vi "SeqLoop.vi"(6 "SEQ STEP Display":refnum<notifier>, 8 "error in (no error)":errorcluster, 9 "SEQ":refnum<queue>, 10 "CORE":refnum<queue>, 11 "WINFAS 2 Data Queue":T1) -> (0 "error out":errorcluster)   [LabVIEW 2014, in "SeqLoop.lvlib"]
uses:
  SeqLoop.lvlib
  APIs/Message Queue/Message Cluster.ctl
  APIs/Data Queue/All Data Queues Cluster.ctl
  APIs/Data Queue/Acquisition Data 1 Sample Cluster.ctl
  APIs/Data Queue/Control Data Cluster.ctl
  APIs/Data Queue/Async Acquisition Data Cluster.ctl
  TypeDefs/STEP Display.ctl
  Mimico Display/TypeDefs/Mimic Data.ctl
  Mimico Display/TypeDefs/BG Image.ctl
  Mimico Display/TypeDefs/mObject.ctl
  TypeDefs/Program.ctl
  TypeDefs/Sequence.ctl
  TypeDefs/STEP.ctl
  TypeDefs/LogicParsedExpression.ctl
  TypeDefs/HW InOut MAP.ctl
  TypeDefs/HW Variables State.ctl
  TypeDefs/STEP State.ctl
  APIs/Message Queue/Enqueue Message (Single).vi
  SEQ Monitoring Global Variables.vi
  APIs/Message Queue/WINFAS 2 Message Queue.lvlib
  Mimico Display/Mimico Display.lvlib
  APIs/Data Queue/WINFAS 2 Data Queue.lvlib
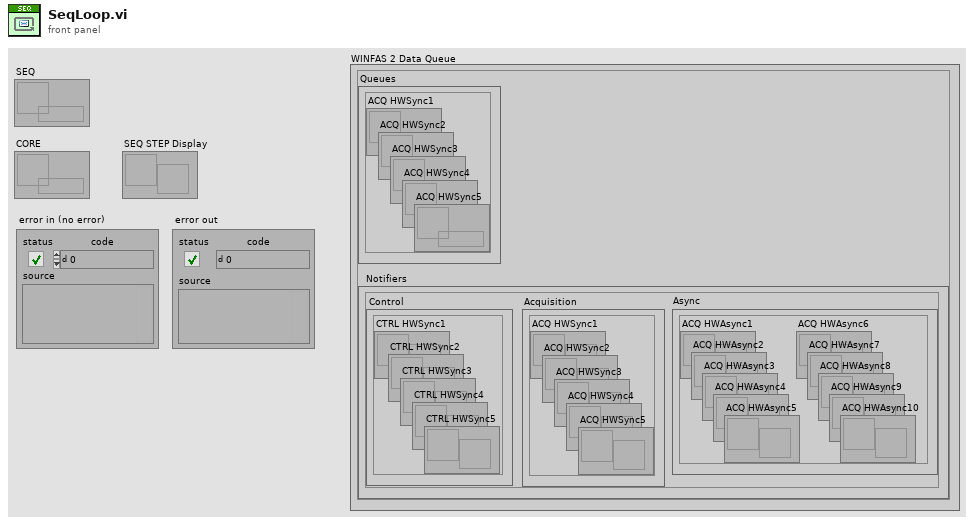
[diagram p1: front panel]
types:
  T1 = typedef "WINFAS 2 Data Queue.lvlib/All Data Queues Cluster.ctl" = cluster{"Queues":cluster{"ACQ HWSync1":refnum<queue>, "ACQ HWSync2":refnum<queue>, "ACQ HWSync3":refnum<queue>, "ACQ HWSync4":refnum<queue>, "ACQ HWSync5":refnum<queue>}, "Notifiers":cluster{"Control":cluster{"CTRL HWSync1":refnum<notifier>, "CTRL HWSync2":refnum<notifier>, "CTRL HWSync3":refnum<notifier>, "CTRL HWSync4":refnum<notifier>, "CTRL HWSync5":refnum<notifier>}, "Acquisition":cluster{"ACQ HWSync1":refnum<notifier>, "ACQ HWSync2":refnum<notifier>, "ACQ HWSync3":refnum<notifier>, "ACQ HWSync4":refnum<notifier>, "ACQ HWSync5":refnum<notifier>}, "Async":cluster{"ACQ HWAsync1":refnum<notifier>, "ACQ HWAsync2":refnum<notifier>, "ACQ HWAsync3":refnum<notifier>, "ACQ HWAsync4":refnum<notifier>, "ACQ HWAsync5":refnum<notifier>, "ACQ HWAsync6":refnum<notifier>, "ACQ HWAsync7":refnum<notifier>, "ACQ HWAsync8":refnum<notifier>, "ACQ HWAsync9":refnum<notifier>, "ACQ HWAsync10":refnum<notifier>}}}
  T2 = typedef "SeqLoop.lvlib/Sequence.ctl" = cluster{"STEPs":T3[], "Main Error&Alarm":cluster{"Main Error":T4, "Main Alarm 1":T4, "Main Alarm 2":T4, "Main Alarm 3":T4, "Main Alarm 4":T4}}
  T3 = typedef "SeqLoop.lvlib/STEP.ctl" = cluster{"STEP N°":u32, "STEP Switch":cluster{"jump?":bool, "Initial STEP":u32, "Number of STEPs":u32, "Repetitions":u32, "Reset?":bool}, "Outputs":i32[], "STEP Check":cluster{"Advance":T4, "Error ":T4, "Alarm 1":T4, "Alarm 2":T4, "Alarm 3":T4, "Alarm 4":T4}, "Display":cluster{"Mssg Op":string, "Mimic Data":T5}}
  T4 = typedef "SeqLoop.lvlib/LogicParsedExpression.ctl" = cluster{"RPN ":string[], "Variables":string[], "Ctes":string[], "Formula":string, "Message":string}
  T5 = typedef "SeqLoop.lvlib/Mimico Display.lvlib/Mimic Data.ctl" = cluster{"BG Image":T6, "Mimic mObjects":T7[]}
  T6 = typedef "SeqLoop.lvlib/Mimico Display.lvlib/BG Image.ctl" = cluster{"Path":path, "point":cluster{"x":i16, "y":i16}}
  T7 = typedef "SeqLoop.lvlib/Mimico Display.lvlib/mObject.ctl" = cluster{"point":cluster{"x":i16, "y":i16}, "Precision (Digits)":i32, "Visible?":bool, "Ref":string, "Comment":string}
  T8 = typedef "SeqLoop.lvlib/STEP State.ctl" = enum16{"Stopped", "First Call", "Idle...", "Advance OK", "Alarm", "Output Security", "Error"}
  T9 = typedef "SeqLoop.lvlib/HW Variables State.ctl" = cluster{"I":bool[], "P":bool[], "N":bool[], "T":bool[], "X":bool[], "Timer":u32[], "Wait":u32, "Wait?":bool, "Jump":cluster{"Jumping?":bool, "Previous STEP to Jump":u32, "Initial Jump STEP":u32, "STEP Count":u32, "Loop Count":u32, "Number of STEPs":u32, "Repetitions":u32}, "Reset?":bool}
  T10 = typedef "SeqLoop.lvlib/HW InOut MAP.ctl" = cluster{"Inputs":cluster{"Entrada":i32, "Descripción":string, "Habilitada?":bool}[][], "Outputs":cluster{"Salida":i32, "Descripción":string, "Habilitada?":bool, "Formula":string, "Tipo de Salida":string}[][]}
  T11 = typedef "SeqLoop.lvlib/Program.ctl" = cluster{"Prog. Data":cluster{"Operación":i32, "Pieza":i32, "Descripción":string, "Nombre Programa":string, "Autor":string, "Diseño":string, "Total Meds.:":i32, "Total Meds. Aux.:":i32}, "All Sequences":cluster{"Measurement":T2, "AutoZero":T2}}
  T12 = cluster{"CTRL HWSync1":refnum<notifier>, "CTRL HWSync2":refnum<notifier>, "CTRL HWSync3":refnum<notifier>, "CTRL HWSync4":refnum<notifier>, "CTRL HWSync5":refnum<notifier>}
  T13 = cluster{"File Direction":path, "Progs Data":variant}
  T14 = typedef "SeqLoop.lvlib/HW CTRL Data.ctl" = cluster{"Inputs":bool[], "Encoder 1":sgl, "Encoder 2":sgl, "Encoder 3":sgl, "Encoder 4":sgl, "Encoder 5":sgl}
  T15 = cluster{"Alarm 1":bool, "Alarm 2":bool, "Alarm 3":bool, "Alarm 4":bool, "Main Err&Alarm?":bool}
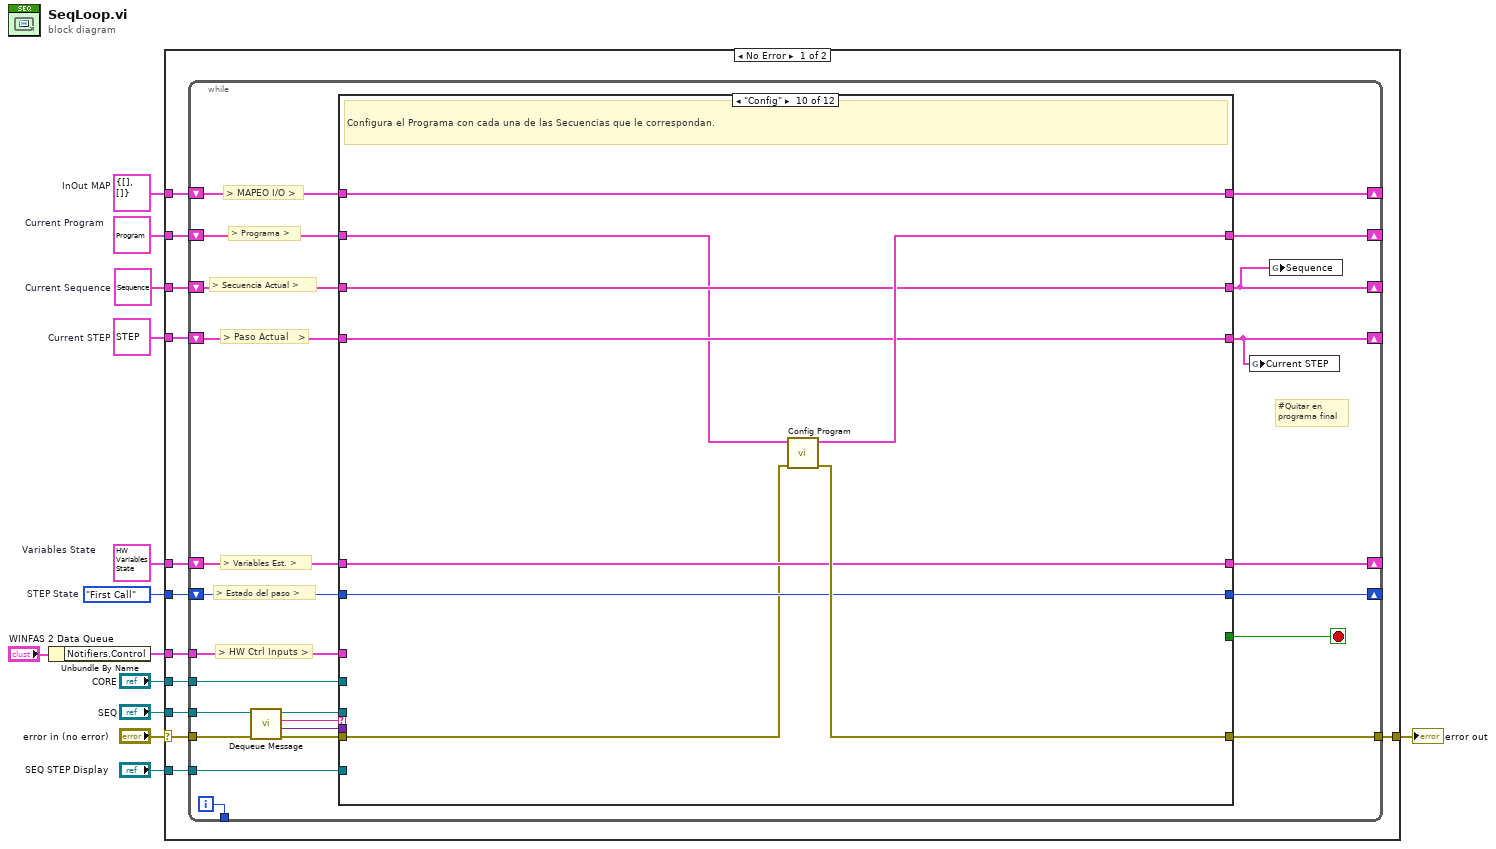
[diagram p0: block diagram]
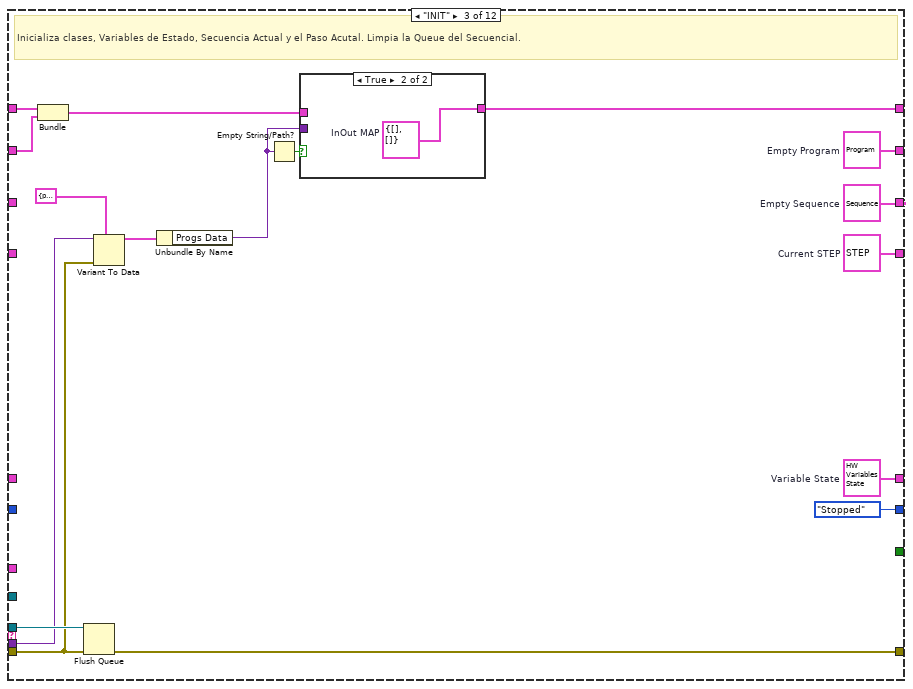
[diagram p4: hidden frame]
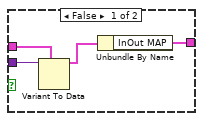
[diagram p5: hidden frame]
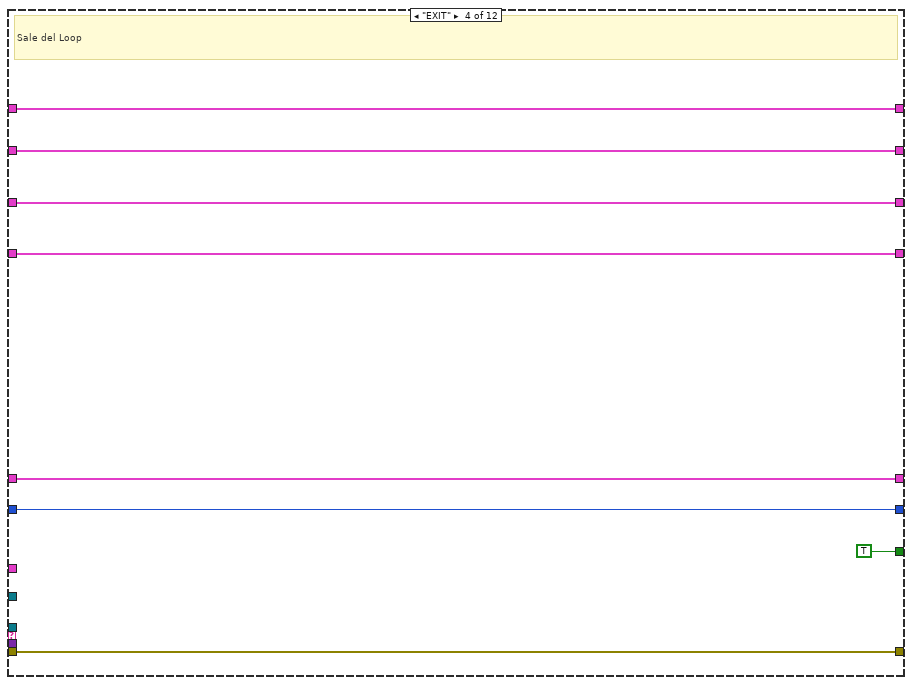
[diagram p6: hidden frame]
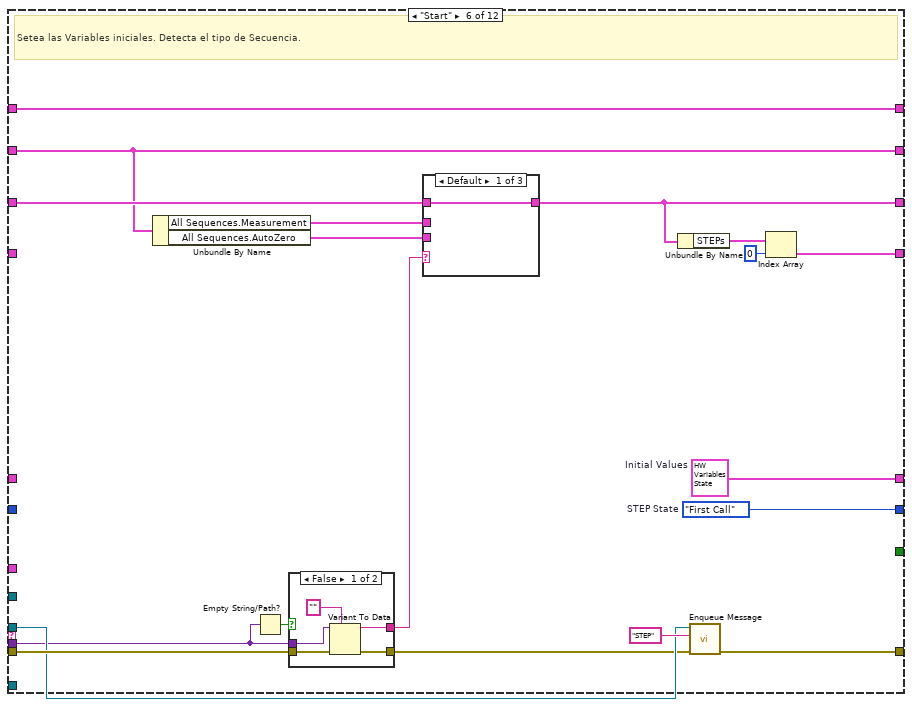
[diagram p8: hidden frame]
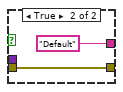
[diagram p9: hidden frame]
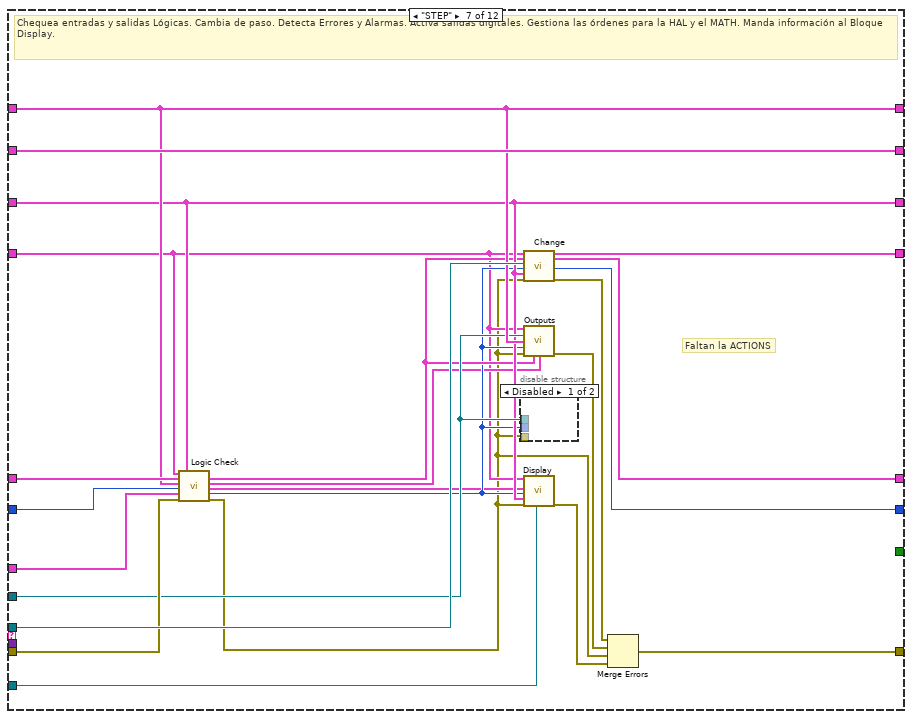
[diagram p12: hidden frame]
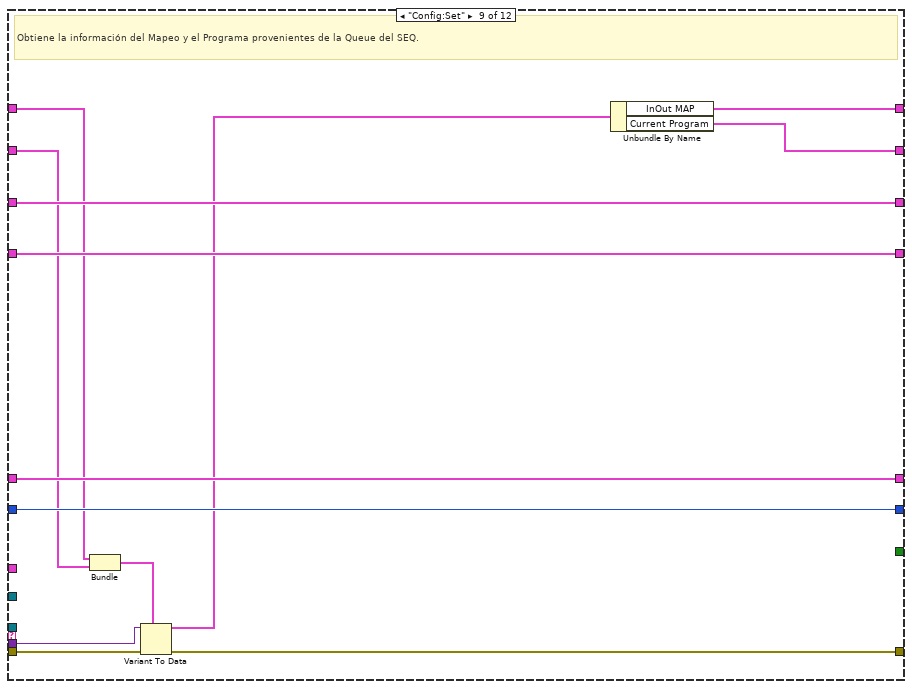
[diagram p15: hidden frame]
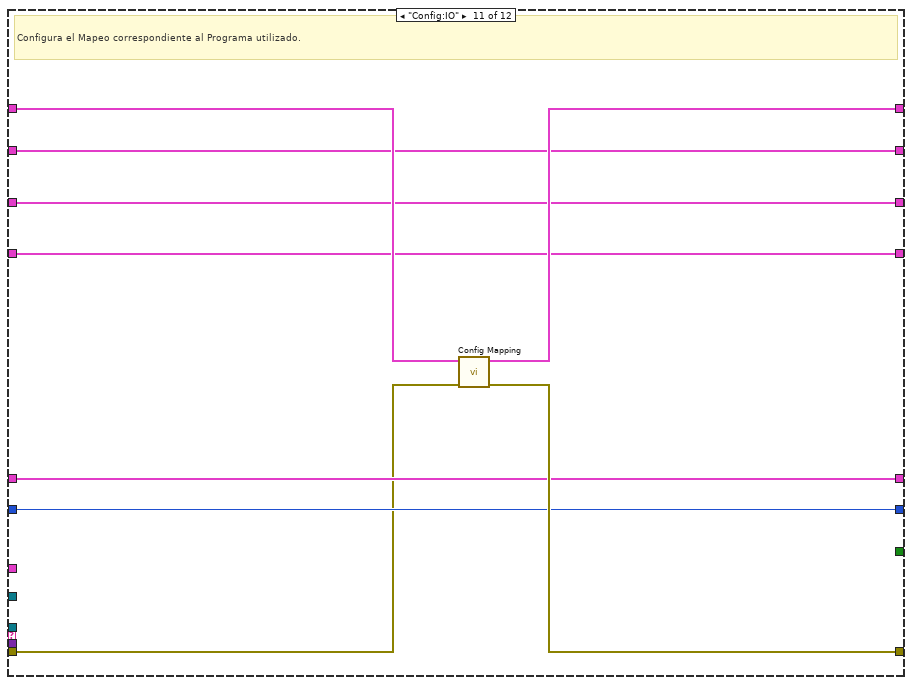
[diagram p16: hidden frame]
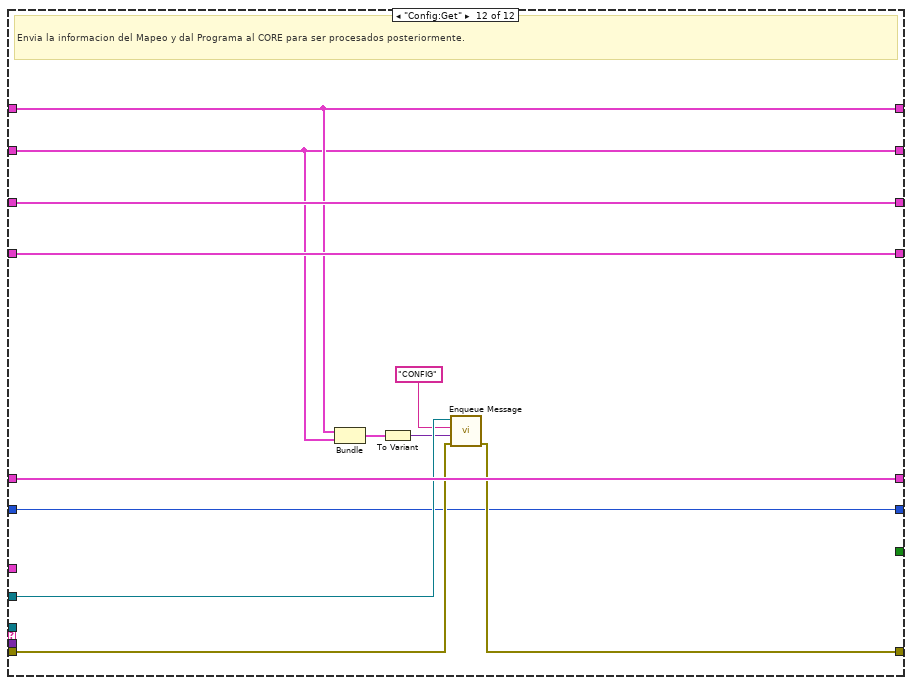
[diagram p17: hidden frame]
diagram:
  w2 = T2 {"STEPs"=[], "Main Error&Alarm"={"Main Error"={"RPN "=[], "Variables"=[], "Ctes"=[], "Formula"="", "Message"=""}, "Main Alarm 1"={"RPN "=[], "Variables"=[], "Ctes"=[], "Formula"="", "Message"=""}, "Main Alarm 2"={"RPN "=[], "Variables"=[], "Ctes"=[], "Formula"="", "Message"=""}, "Main Alarm 3"={"RPN "=[], "Variables"=[], "Ctes"=[], "Formula"="", "Message"=""}, "Main Alarm 4"={"RPN "=[], "Variables"=[], "Ctes"=[], "Formula"="", "Message"=""}}}  # Current Sequence
  w1 = T3 {"STEP N°"=0, "STEP Switch"={"jump?"=FALSE, "Initial STEP"=0, "Number of STEPs"=0, "Repetitions"=0, "Reset?"=FALSE}, "Outputs"=[], "STEP Check"={"Advance"={"RPN "=[], "Variables"=[], "Ctes"=[], "Formula"="", "Message"=""}, "Error "={"RPN "=[], "Variables"=[], "Ctes"=[], "Formula"="", "Message"=""}, "Alarm 1"={"RPN "=[], "Variables"=[], "Ctes"=[], "Formula"="", "Message"=""}, "Alarm 2"={"RPN "=[], "Variables"=[], "Ctes"=[], "Formula"="", "Message"=""}, "Alarm 3"={"RPN "=[], "Variables"=[], "Ctes"=[], "Formula"="", "Message"=""}, "Alarm 4"={"RPN "=[], "Variables"=[], "Ctes"=[], "Formula"="", "Message"=""}}, "Display"={"Mssg Op"="", "Mimic Data"={"BG Image"={"Path"=path "", "point"={"x"=0, "y"=0}}, "Mimic mObjects"=[]}}}  # Current STEP
  w6 = STEP_State."First Call"  # STEP State
  w7 = T9 {"I"=[], "P"=[], "N"=[], "T"=[], "X"=[], "Timer"=[], "Wait"=0, "Wait?"=FALSE, "Jump"={"Jumping?"=FALSE, "Previous STEP to Jump"=0, "Initial Jump STEP"=0, "STEP Count"=0, "Loop Count"=0, "Number of STEPs"=0, "Repetitions"=0}, "Reset?"=FALSE}  # Variables State
  w9 = T10 {"Inputs"=[], "Outputs"=[]}  # InOut MAP
  w8 = T11 {"Prog. Data"={"Operación"=0, "Pieza"=0, "Descripción"="", "Nombre Programa"="", "Autor"="", "Diseño"="", "Total Meds.:"=0, "Total Meds. Aux.:"=0}, "All Sequences"={"Measurement"={"STEPs"=[], "Main Error&Alarm"={"Main Error"={"RPN "=[], "Variables"=[], "Ctes"=[], "Formula"="", "Message"=""}, "Main Alarm 1"={"RPN "=[], "Variables"=[], "Ctes"=[], "Formula"="", "Message"=""}, "Main Alarm 2"={"RPN "=[], "Variables"=[], "Ctes"=[], "Formula"="", "Message"=""}, "Main Alarm 3"={"RPN "=[], "Variables"=[], "Ctes"=[], "Formula"="", "Message"=""}, "Main Alarm 4"={"RPN "=[], "Variables"=[], "Ctes"=[], "Formula"="", "Message"=""}}}, "AutoZero"={"STEPs"=[], "Main Error&Alarm"={"Main Error"={"RPN "=[], "Variables"=[], "Ctes"=[], "Formula"="", "Message"=""}, "Main Alarm 1"={"RPN "=[], "Variables"=[], "Ctes"=[], "Formula"="", "Message"=""}, "Main Alarm 2"={"RPN "=[], "Variables"=[], "Ctes"=[], "Formula"="", "Message"=""}, "Main Alarm 3"={"RPN "=[], "Variables"=[], "Ctes"=[], "Formula"="", "Message"=""}, "Main Alarm 4"={"RPN "=[], "Variables"=[], "Ctes"=[], "Formula"="", "Message"=""}}}}}  # Current Program
  n1 = Unbundle By Name("WINFAS 2 Data Queue") -> ("Notifiers.Control"=w4:T12)
  n2 = case shown="No Error" "error in (no error)" {
    selector: "error in (no error)" -> [w25 w203]
    tunnel: [w18 w203] -> w12
    tunnel: "CORE" -> [w24 _]
    tunnel: "SEQ" -> [w23 _]
    tunnel: w9 -> [w22 _]
    tunnel: w8 -> [w21 _]
    tunnel: w2 -> [w17 _]
    tunnel: w7 -> [w20 _]
    tunnel: "SEQ STEP Display" -> [w19 _]
    tunnel: w6 -> [w16 _]
    tunnel: w4 -> [w15 _]
    tunnel: w1 -> [w14 _]
    frame No Error {
      n3 = while {
        tunnel: w25 -> [w45]
        tunnel: [w33] -> w18
        tunnel: w23 -> [w46]
        shift-right: [w47] -> _
        shift-left: w20 -> [w48]
        shift-right: [w40] -> _
        shift-left: w22 -> [w41]
        shift-right: [w38] -> _
        shift-left: w21 -> [w39]
        tunnel: w24 -> [w37]
        tunnel: w19 -> [w36]
        shift-right: [w28] -> _
        shift-left: w17 -> [w34]
        tunnel: w15 -> [w35]
        shift-right: [w26] -> _
        shift-left: w14 -> [w30]
        shift-right: [w29] -> _
        shift-left: w16 -> [w31]
        tunnel: [w27] -> _
        i -> [w27]
        stop <- w49 stop-if-true
        # "#Quitar en\nprograma final"
        # "> HW Ctrl Inputs >"
        # "> Variables Est. >"
        # "> Estado del paso >"
        # "> Paso Actual   >"
        # "> Secuencia Actual >"
        # "> Programa >"
        # "> MAPEO I/O >"
        n4 = call "Dequeue Message.vi"("error in (no error)"=w45, "Message Queue"=w46) -> ("error out"=w44:errorcluster, "Message Data"=w42:variant, "Message"=w43:string, "dup Message Queue"=w32:refnum<queue>)  [unwired: 6 in]
        n5 = case shown="\"Config\"" w43 {
          tunnel: [w55 w59 w78 w91 w100 w111 w147 w158 w161 w181 w190 w199] -> w33
          tunnel: w44 -> [w55 w59 w76 w91 w100 w117 w142 w158 w171 w174 w182 w200]
          tunnel: w42 -> [_ _ w75 _ _ w102 _ _ w170 _ _ _]
          tunnel: [_ _ _ TRUE _ _ _ _ _ _ _ _] -> w49
          tunnel: w48 -> [w56 w63 _ w92 w99 _ w145 w159 w172 w180 w189 w202]
          tunnel: [w56 w63 w79 w92 w99 w109 w137 w159 w172 w180 w189 w202] -> w47
          tunnel: w41 -> [w52 w61 w72 w88 w97 w115 w141 w155 w164 w179 w188 w193]
          tunnel: [w52 w61 w70 w88 w97 w115 w141 w155 w167 w179 w187 w193] -> w40
          tunnel: w39 -> [w54 w62 w71 w90 w98 w112 w150 w157 w163 w173 w186 w192]
          tunnel: [w54 w62 w65 w90 w98 w112 w150 w157 w168 w178 w186 w192] -> w38
          tunnel: w37 -> [_ _ _ _ _ _ w140 _ _ _ _ w201]
          tunnel: w36 -> [_ _ _ _ _ _ w144 _ _ _ _ _]
          tunnel: [w53 w60 w64 w89 w96 w105 w136 w156 w169 w177 w185 w197] -> w28
          tunnel: w34 -> [w53 w60 _ w89 w96 w113 w136 w156 w169 w177 w185 w197]
          tunnel: w35 -> [_ _ _ _ _ _ w146 _ _ _ _ _]
          tunnel: w32 -> [_ _ w80 _ _ w114 w148 _ _ _ _ _]
          tunnel: w31 -> [w50 w57 _ w86 w94 _ w143 w153 w165 w175 w183 w195]
          tunnel: [w51 w58 w67 w87 w95 w103 w151 w154 w166 w176 w184 w196] -> w26
          tunnel: w30 -> [w51 w58 _ w87 w95 _ w131 w154 w166 w176 w184 w196]
          tunnel: [w50 w57 STEP_State."Stopped" ("STEP State") w86 w94 w107 w149 w153 w165 w175 w183 w195] -> w29
          frame "----LOOP----" {
            # "Bloque que adminte futuras configuraciones al inicio."
          }
          frame Default {
          }
          frame "INIT" {
            w64 = T2 {"STEPs"=[], "Main Error&Alarm"={"Main Error"={"RPN "=[], "Variables"=[], "Ctes"=[], "Formula"="", "Message"=""}, "Main Alarm 1"={"RPN "=[], "Variables"=[], "Ctes"=[], "Formula"="", "Message"=""}, "Main Alarm 2"={"RPN "=[], "Variables"=[], "Ctes"=[], "Formula"="", "Message"=""}, "Main Alarm 3"={"RPN "=[], "Variables"=[], "Ctes"=[], "Formula"="", "Message"=""}, "Main Alarm 4"={"RPN "=[], "Variables"=[], "Ctes"=[], "Formula"="", "Message"=""}}}  # Empty Sequence
            w67 = T3 {"STEP N°"=0, "STEP Switch"={"jump?"=FALSE, "Initial STEP"=0, "Number of STEPs"=0, "Repetitions"=0, "Reset?"=FALSE}, "Outputs"=[], "STEP Check"={"Advance"={"RPN "=[], "Variables"=[], "Ctes"=[], "Formula"="", "Message"=""}, "Error "={"RPN "=[], "Variables"=[], "Ctes"=[], "Formula"="", "Message"=""}, "Alarm 1"={"RPN "=[], "Variables"=[], "Ctes"=[], "Formula"="", "Message"=""}, "Alarm 2"={"RPN "=[], "Variables"=[], "Ctes"=[], "Formula"="", "Message"=""}, "Alarm 3"={"RPN "=[], "Variables"=[], "Ctes"=[], "Formula"="", "Message"=""}, "Alarm 4"={"RPN "=[], "Variables"=[], "Ctes"=[], "Formula"="", "Message"=""}}, "Display"={"Mssg Op"="", "Mimic Data"={"BG Image"={"Path"=path "", "point"={"x"=0, "y"=0}}, "Mimic mObjects"=[]}}}  # Current STEP
            w65 = T11 {"Prog. Data"={"Operación"=0, "Pieza"=0, "Descripción"="", "Nombre Programa"="", "Autor"="", "Diseño"="", "Total Meds.:"=0, "Total Meds. Aux.:"=0}, "All Sequences"={"Measurement"={"STEPs"=[], "Main Error&Alarm"={"Main Error"={"RPN "=[], "Variables"=[], "Ctes"=[], "Formula"="", "Message"=""}, "Main Alarm 1"={"RPN "=[], "Variables"=[], "Ctes"=[], "Formula"="", "Message"=""}, "Main Alarm 2"={"RPN "=[], "Variables"=[], "Ctes"=[], "Formula"="", "Message"=""}, "Main Alarm 3"={"RPN "=[], "Variables"=[], "Ctes"=[], "Formula"="", "Message"=""}, "Main Alarm 4"={"RPN "=[], "Variables"=[], "Ctes"=[], "Formula"="", "Message"=""}}}, "AutoZero"={"STEPs"=[], "Main Error&Alarm"={"Main Error"={"RPN "=[], "Variables"=[], "Ctes"=[], "Formula"="", "Message"=""}, "Main Alarm 1"={"RPN "=[], "Variables"=[], "Ctes"=[], "Formula"="", "Message"=""}, "Main Alarm 2"={"RPN "=[], "Variables"=[], "Ctes"=[], "Formula"="", "Message"=""}, "Main Alarm 3"={"RPN "=[], "Variables"=[], "Ctes"=[], "Formula"="", "Message"=""}, "Main Alarm 4"={"RPN "=[], "Variables"=[], "Ctes"=[], "Formula"="", "Message"=""}}}}}  # Empty Program
            w79 = T9 {"I"=[], "P"=[], "N"=[], "T"=[], "X"=[], "Timer"=[], "Wait"=0, "Wait?"=FALSE, "Jump"={"Jumping?"=FALSE, "Previous STEP to Jump"=0, "Initial Jump STEP"=0, "STEP Count"=0, "Loop Count"=0, "Number of STEPs"=0, "Repetitions"=0}, "Reset?"=FALSE}  # Variable State
            # "Inicializa clases, Variables de Estado, Secuencia Actual y el Paso Acutal. Limpia la Queue del Secuencial."
            n6 = Bundle("InOut MAP"=w72, "Current Program"=w71) -> (w73:cluster{"InOut MAP":T10, "Current Program":T11})  [unwired: 1 in]
            n7 = Flush Queue(queue=w80, error in (no error)=w76) -> (error out=w78:errorcluster)  [unwired: 2 out]
            n8 = Variant To Data(error in=w76, type=T13 {"File Direction"=path "", "Progs Data"=variant} ("element"), Variant=w75) -> (data=w74:T13)  [unwired: 1 out]
            n9 = Unbundle By Name(w74) -> ("Progs Data"=w69:variant)
            n10 = Empty String/Path?(string/path=w69) -> (empty?=w68:bool)
            n11 = case shown="True" w68 {
              tunnel: w73 -> [w84 _]
              tunnel: [w82 w85] -> w70
              tunnel: w69 -> [w81 _]
              frame False {
                n12 = Variant To Data(type=w84, Variant=w81) -> (data=w83:cluster{"InOut MAP":T10, "Current Program":T11})  [unwired: 1 in, 1 out]
                n13 = Unbundle By Name(w83) -> ("InOut MAP"=w82:T10)
              }
              frame True {
                w85 = T10 {"Inputs"=[], "Outputs"=[]}  # InOut MAP
              }
            }
          }
          frame "EXIT" {
            # "Sale del Loop"
          }
          frame "----ACTION----" {
          }
          frame "Start" {
            w107 = STEP_State."First Call"  # STEP State
            w109 = T9 {"I"=[], "P"=[], "N"=[], "T"=[], "X"=[], "Timer"=[], "Wait"=0, "Wait?"=FALSE, "Jump"={"Jumping?"=FALSE, "Previous STEP to Jump"=0, "Initial Jump STEP"=0, "STEP Count"=0, "Loop Count"=0, "Number of STEPs"=0, "Repetitions"=0}, "Reset?"=FALSE}  # Initial Values
            # "Setea las Variables iniciales. Detecta el tipo de Secuencia."
            n14 = Unbundle By Name(w112) -> ("All Sequences.Measurement"=w119:T2, "All Sequences.AutoZero"=w118:T2)
            n15 = Empty String/Path?(string/path=w102) -> (empty?=w101:bool)
            n16 = case shown="False" w101 {
              tunnel: w117 -> [w124 w126]
              tunnel: [w122 "Default"] -> w110
              tunnel: [w121 w126] -> w106
              tunnel: w102 -> [w120 _]
              frame False {
                n17 = Variant To Data(error in=w124, type="", Variant=w120) -> (data=w122:string, error out=w121:errorcluster)
              }
              frame True {
              }
            }
            n18 = case shown="Default" w110 {
              tunnel: w119 -> [_ w128 _]
              tunnel: w118 -> [_ _ w129]
              tunnel: [w127 w128 w129] -> w105
              tunnel: w113 -> [w127 _ _]
              frame Default {
              }
              frame "Measurement" {
              }
              frame "Auto-Zero" {
              }
            }
            n19 = Unbundle By Name(w105) -> ("STEPs"=w104:T3[])
            n20 = call-poly "Enqueue Message.vi"("error in (no error)"=w106, "Message"="STEP", "Message Queue"=w114) -> ("error out"=w111:errorcluster)  [unwired: 7 in, 1 out]
            n21 = Index Array(array=w104, index=0) -> (element=w103:T3)
          }
          frame "STEP" {
            # "Faltan la ACTIONS"
            # "Chequea entradas y salidas Lógicas. Cambia de paso. Detecta Errores y Alarmas. Activa salidas digitales. Gestiona las órdenes para la HAL y el MATH. Manda información al Bloque Display."
            n22 = call "Logic Check.vi"("STEP in"=w131, "Variables State in"=w145, "HW InOut MAP"=w141, "STEP State in"=w143, "Notifiers.Control"=w146, "error in (no error)"=w142, "Current Sequence"=w136) -> ("Variables State out"=w135:T9, "HW CTRL Data"=w132:T14, "Alarms triggered?"=w133:T15, "STEP State out"=w134:T8, "error out"=w130:errorcluster)  [unwired: 7 in, 1 out]
            n23 = disable-structure shown="Disabled" {
              disable-tunnel: w140 -> [_ _]
              disable-tunnel: w130 -> [_ _]
              disable-tunnel: w134 -> [_ _]
              frame Disabled {
              }
              frame Enabled {
              }
            }
            n24 = call "Change.vi"("STEP"=w131, "Variables State"=w135, "SEQ"=w148, "STEP State"=w134, "Current Sequence"=w136, "error in (no error)"=w130) -> ("STEP Out"=w151:T3, "Variables State out"=w137:T9, "STEP State out"=w149:T8, "error out"=w139:errorcluster)  [unwired: 10 in]
            n25 = call "Outputs.vi"("STEP in"=w131, "CORE"=w140, "Mapping Buss"=w141, "STEP State"=w134, "error in (no error)"=w130, "Variables State in"=w135, "HW CTRL Data"=w132) -> ("error out"=w138:errorcluster)  [unwired: 7 in, 1 out]
            n26 = call "Display.vi"("STEP in"=w131, "Alarms triggered?"=w133, "STEP State"=w134, "Current Sequence"=w136, "error in (no error)"=w130, "SEQ STEP Display"=w144) -> ("error out"=w152:errorcluster)  [unwired: 12 in, 1 out]
            n27 = Merge Errors(w139, w138, w130, w152) -> (w147:errorcluster)
          }
          frame "----UTILITY----" {
          }
          frame "Config:Set" {
            # "Obtiene la información del Mapeo y el Programa provenientes de la Queue del SEQ."
            n28 = Bundle("InOut MAP"=w164, "Current Program"=w163) -> (w162:cluster{"InOut MAP":T10, "Current Program":T11})  [unwired: 1 in]
            n29 = Variant To Data(error in=w171, type=w162, Variant=w170) -> (data=w160:cluster{"InOut MAP":T10, "Current Program":T11}, error out=w161:errorcluster)
            n30 = Unbundle By Name(w160) -> ("InOut MAP"=w167:T10, "Current Program"=w168:T11)
          }
          frame "Config" {
            # "Configura el Programa con cada una de las Secuencias que le correspondan."
            n31 = call "Config Program.vi"("error in (no error)"=w174, "Prog in"=w173) -> ("error out"=w181:errorcluster, "Prog out"=w178:T11)  [unwired: 8 in]
          }
          frame "Config:IO" {
            # "Configura el Mapeo correspondiente al Programa utilizado."
            n32 = call "Config Mapping.vi"("error in (no error)"=w182, "HW InOut MAP in"=w188) -> ("error out"=w190:errorcluster, "HW InOut MAP out"=w187:T10)  [unwired: 8 in]
          }
          frame "Config:Get" {
            # "Envia la informacion del Mapeo y dal Programa al CORE para ser procesados posteriormente."
            n33 = Bundle("InOut MAP"=w193, "Current Program"=w192) -> (w191:cluster{"InOut MAP":T10, "Current Program":T11})  [unwired: 1 in]
            n34 = To Variant(anything=w191) -> (Variant=w194:variant)
            n35 = call-poly "Enqueue Message.vi"("error in (no error)"=w200, "Message Data"=w194, "Message"="CONFIG", "Message Queue"=w201) -> ("error out"=w199:errorcluster)  [unwired: 6 in, 1 out]
          }
        }
        n36 = global write "SEQ Monitoring Global Variables.vi" "Current STEP"(w26) -> ()
        n37 = global write "SEQ Monitoring Global Variables.vi" "Sequence"(w28) -> ()
      }
    }
    frame Error {
    }
  }
  "error out" <- w12
